vi "Check and Toggle Error.vi"(4 "error string":string, 6 "error key":string, 8 "error In":errorcluster, 9 "error code":i32, 10 "clear error":bool, 11 "item reference in":T1 format="%.0x") -> (0 "error out":errorcluster, 3 "item reference out":T1 format="%.0x")   [LabVIEW 2027, in "Embedded Data Logger System Explorer.lvlib"]
doc: "Adds or removes an error from VeriStand's system definition central error handler."
uses:
  Embedded Data Logger System Explorer.lvlib
  <vilib>/NI VeriStand/Custom Device API/Custom Device Item Ref.ctl
  <vilib>/NI/NI VeriStand Error API/VeriStand Error.ctl
  <vilib>/NI/NI VeriStand Error API/VeriStand Error API.lvlib
  <vilib>/NI VeriStand/Custom Device API/Custom Device API.lvlib
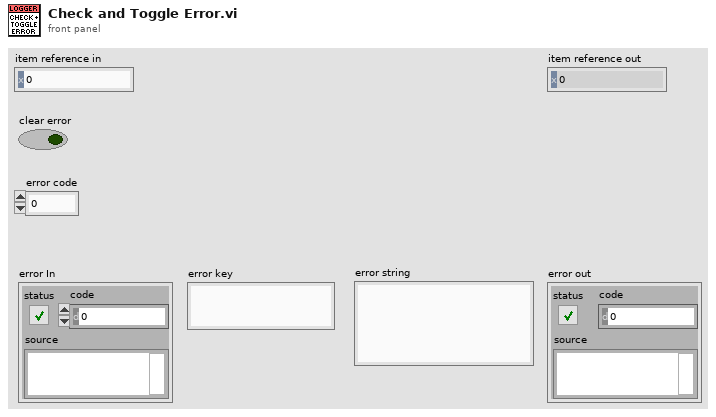
[diagram p1: front panel]
types:
  T1 = typedef "Custom Device API.lvlib/Custom Device Item Ref.ctl" = u64
  T2 = typedef "VeriStand Error API.lvlib/VeriStand Error.ctl" = cluster{"status":bool, "code":i32, "message":string}
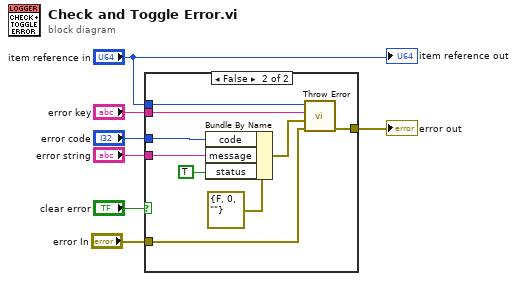
[diagram p0: block diagram]
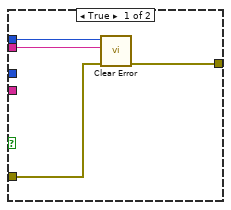
[diagram p2: hidden frame]
diagram:
  n1 = case shown="False" "clear error" {
    tunnel: "error string" -> [_ w16]
    tunnel: "item reference in" -> [w11 w20]
    tunnel: "error key" -> [w10 w19]
    tunnel: "error code" -> [_ w17]
    tunnel: "error In" -> [w9 w13]
    tunnel: [w8 w12] -> w1
    frame True {
      n2 = call <vilib>:"Clear Error.vi"("error in (no error)"=w9, "Key"=w10, "Item Ref in"=w11) -> ("error out"=w8:errorcluster)  [unwired: 7 in, 1 out]
    }
    frame False {
      n3 = Bundle By Name(cluster=T2 {"status"=FALSE, "code"=0, "message"=""} ("VeriStand Error In"), "code"=w17, "message"=w16, "status"=TRUE) -> (w14:T2)
      n4 = call <vilib>:"Throw Error.vi"("error in"=w13, "VeriStand Error In"=w14, "Key"=w19, "Item Ref in"=w20) -> ("error out"=w12:errorcluster)  [unwired: 6 in, 1 out]
    }
  }
  "error out" <- w1
  "item reference out" <- "item reference in"
